vi "Read disconnected.vi"(8 "error in (no error)":errorcluster, 11 "Car in":refnum<class "Car.lvclass">) -> (0 "error out":errorcluster, 2 "disconnected":bool, 3 "Car out":refnum<class "Car.lvclass">)   [LabVIEW 2017, in "Car.lvclass"]
uses:
  Car.lvclass
  Car.lvclass/Car.ctl
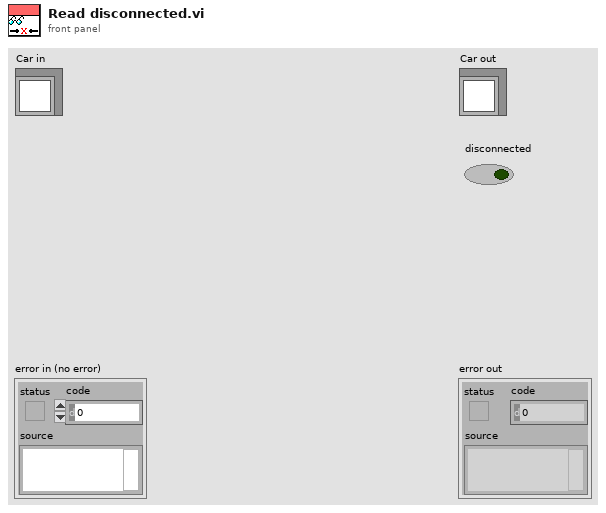
[diagram p1: front panel]
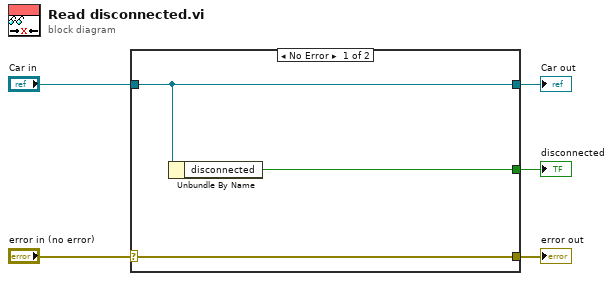
[diagram p0: block diagram]
diagram:
  n1 = case shown="No Error" "error in (no error)" {
    selector: "error in (no error)" -> [w8 w9]
    tunnel: [w8 w9] -> w4
    tunnel: [w7 w10] -> w2
    tunnel: "Car in" -> [w7 w10]
    tunnel: [w6 _] -> w1
    frame No Error {
      n2 = Unbundle By Name(w7) -> ("disconnected"=w6:bool)
    }
    frame Error {
    }
  }
  "error out" <- w4
  "Car out" <- w2
  "disconnected" <- w1
